vi "mSec wait.vi"(8 "Error in":errorcluster, 11 "mSec wait":u32) -> (0 "Error out":errorcluster)   [LabVIEW 2021]
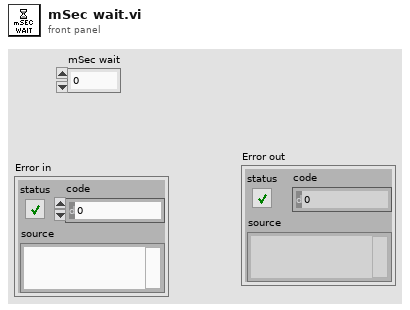
[diagram p1: front panel]
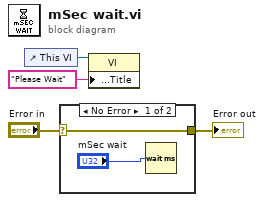
[diagram p0: block diagram]
diagram:
  n1 = control-ref of="This VI"() -> (w2:refnum<vi>)
  n2 = case shown="No Error" "Error in" {
    selector: "Error in" -> [w5 w7]
    tunnel: [w5 w7] -> w3
    frame No Error {
      n3 = Wait (ms)(milliseconds to wait="mSec wait") -> ()  [unwired: 1 out]
    }
    frame Error {
    }
  }
  "Error out" <- w3
  n4 = property class="VI"(reference=w2, "Front Panel.Title"="Please Wait" ("Front Panel Window:Title")) -> ()  [unwired: 1 in, 2 out]
